vi "Insert Calibration into dB.vi"(8 "error in (no error)":errorcluster, 11 "C&C Data In":T1={"Hardware Configuration"={"COM Port"="", "Reference Distance"=0.0, "Sensor SN"=""}, "Logging Configuration"={"Log File Base Path"=path "", "Datafile Ref"=refnum, "Database Ref"=refnum}, "UI Refs"={"Start Ref"=refnum, "Settings Ref"=refnum, "Stop Ref"=refnum, "Exit Ref"=refnum, "Status Ref"=refnum, "Data Ref"=refnum, "StatusBox Ref"=refnum, "Location Ref"=refnum, "Operator Ref"=refnum, "Time Ref"=refnum, "Test in Progess Ref"=refnum}, "Calibration Data"={"calibrationID"=0, "operatorID"=0, "sensorID"=0, "start_time"="", "end_time"="", "offset"=0.0, "offset_units"="", "ring_time"=0.0, "error"=0.0, "Passed"=0, "data_storage_location"="", "comments"=""}, "Time Elapsed"=0, "Samples Required"=480} {"Hardware Configuration"."Reference Distance" format="%.3g"}) -> (0 "error out":errorcluster)   [LabVIEW 2018, in "Logging.lvlib"]
uses:
  Logging.lvlib
  Settings/Settings.ctl
  Acquisition/Hardware Configuration.ctl
  Logging Configuration.ctl
  <vilib>/addons/database/Connection.llb/Conn ObjectReference.ctl
  Controls/Location Ring.ctl
  Controls/Time Remaining.ctl
  OSTEP_MySQLdBTools/MySQLTools.lvlib
  Acquisition/Acquisition.lvlib
  <vilib>/addons/database/NI_Database_API.lvlib
  Settings/Settings.lvlib
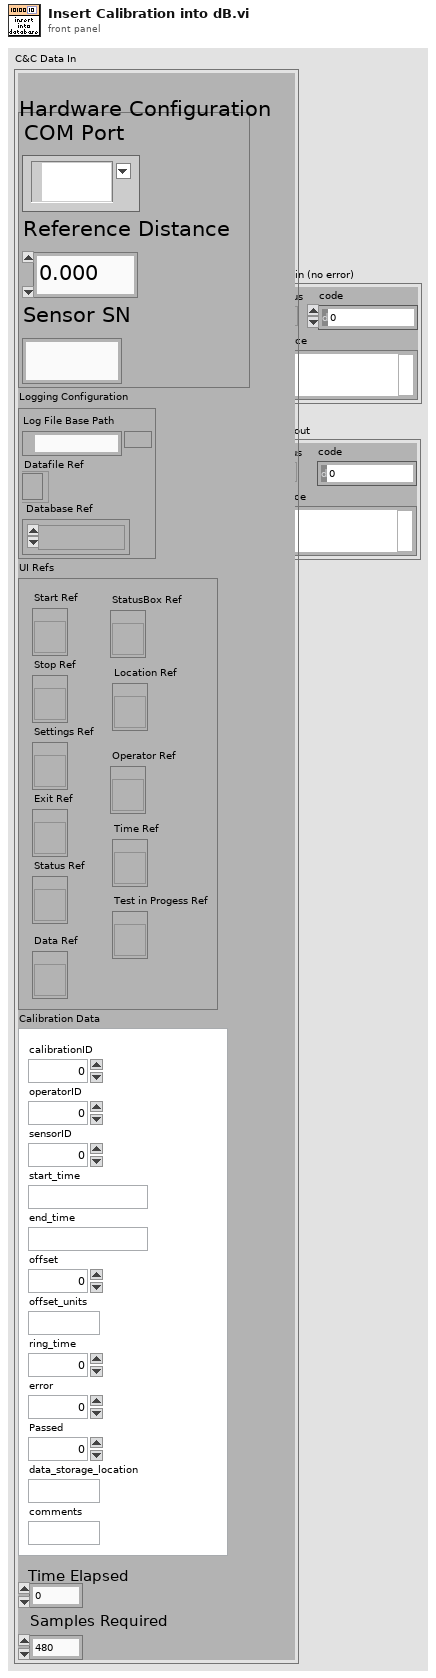
[diagram p1: front panel]
types:
  T1 = typedef "Settings.lvlib/Settings.ctl" = cluster{"Hardware Configuration":T2, "Logging Configuration":T3, "UI Refs":cluster{"Start Ref":refnum<vi>, "Settings Ref":refnum<vi>, "Stop Ref":refnum<vi>, "Exit Ref":refnum<vi>, "Status Ref":refnum<vi>, "Data Ref":refnum<vi>, "StatusBox Ref":refnum<vi>, "Location Ref":refnum<vi>, "Operator Ref":refnum<vi>, "Time Ref":refnum<vi>, "Test in Progess Ref":refnum<vi>}, "Calibration Data":cluster{"calibrationID":u16, "operatorID":u16, "sensorID":u16, "start_time":string, "end_time":string, "offset":dbl, "offset_units":string, "ring_time":dbl, "error":dbl, "Passed":u8, "data_storage_location":string, "comments":string}, "Time Elapsed":u16, "Samples Required":u16}
  T2 = typedef "Acquisition.lvlib/Hardware Configuration.ctl" = cluster{"COM Port":refnum<visa-resource-name>, "Reference Distance":dbl, "Sensor SN":string}
  T3 = typedef "Logging.lvlib/Logging Configuration.ctl" = cluster{"Log File Base Path":path, "Datafile Ref":refnum<file>, "Database Ref":T4}
  T4 = typedef "NI_Database_API.lvlib/Conn ObjectReference.ctl" = refnum<k1>
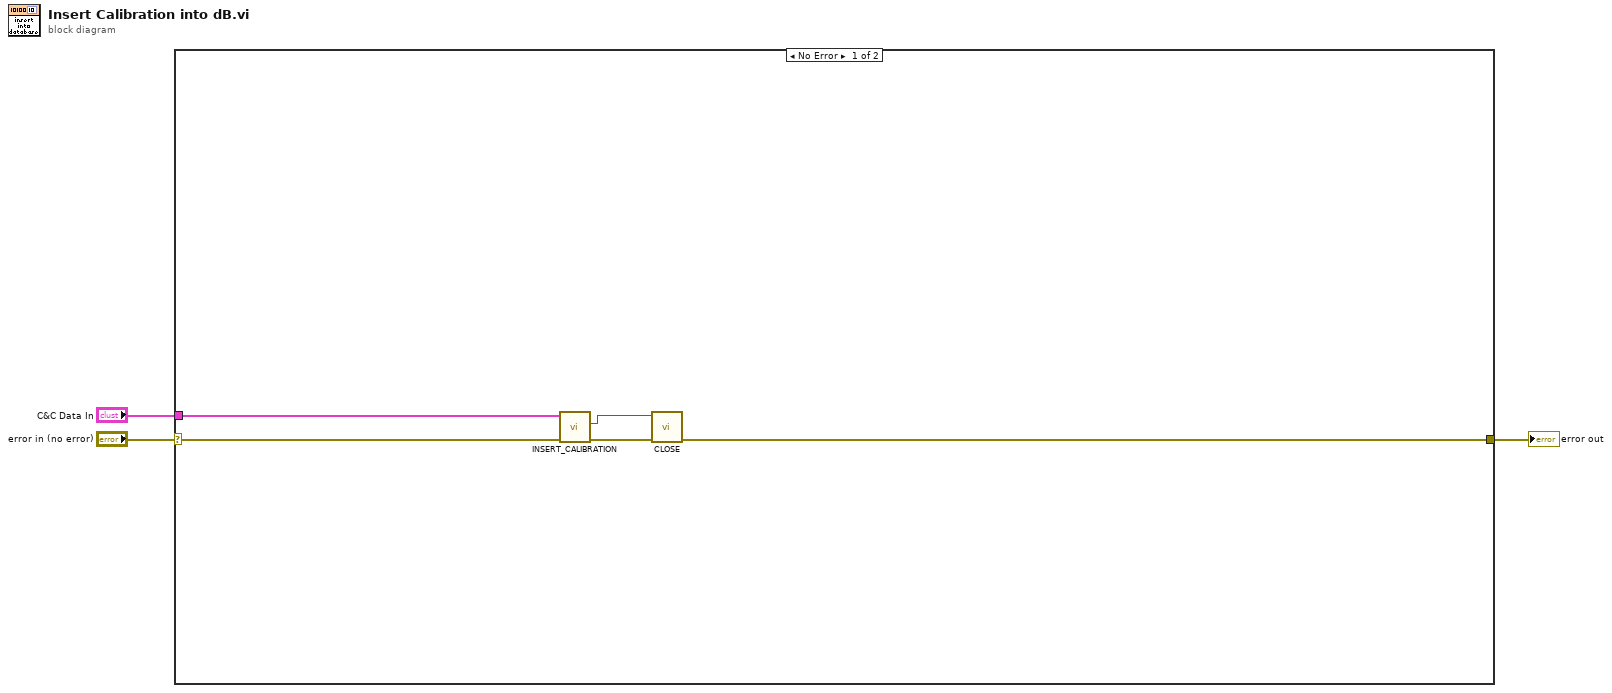
[diagram p0: block diagram]
diagram:
  n1 = case shown="No Error" "error in (no error)" {
    selector: "error in (no error)" -> [w6 w9]
    tunnel: [w4 w9] -> w3
    tunnel: "C&C Data In" -> [w5 _]
    frame No Error {
      n2 = call "INSERT_CALIBRATION.vi"("error in (no error)"=w6, "C&C Data in"=w5) -> ("error out"=w7:errorcluster, "connection reference out"=w8:T4)  [unwired: 8 in]
      n3 = call "CLOSE.vi"("error in (no error)"=w7, "Database Ref In"=w8) -> ("error out"=w4:errorcluster)  [unwired: 9 in]
    }
    frame Error {
    }
  }
  "error out" <- w3
